vi "Write Core.vi"(8 "error in (no error)":errorcluster, 10 "Core":T1, 11 "ModuleAbstract in":refnum<class "ModuleAbstract.lvclass">) -> (0 "error out":errorcluster, 3 "ModuleAbstract out":refnum<class "ModuleAbstract.lvclass">)   [LabVIEW 2019, in "ModuleAbstract.lvlib" / "ModuleAbstract.lvclass"]
uses:
  ModuleAbstract.lvclass
  <vilib>/ActorFramework/Message Enqueuer/Message Enqueuer.lvclass
  ModuleAbstract.lvclass/ModuleAbstract.ctl
  Containers/ActorRefContainer/ActorRefContainer.lvclass/ActorRefContainer.ctl
  Containers/ActorRefContainer/ActorRefContainer.lvclass
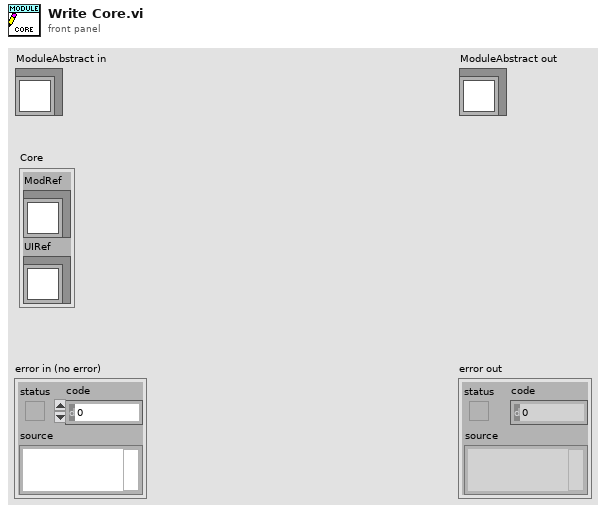
[diagram p1: front panel]
types:
  T1 = cluster{"ModRef":refnum<class "Message Enqueuer.lvclass">, "UIRef":refnum<class "Message Enqueuer.lvclass">}
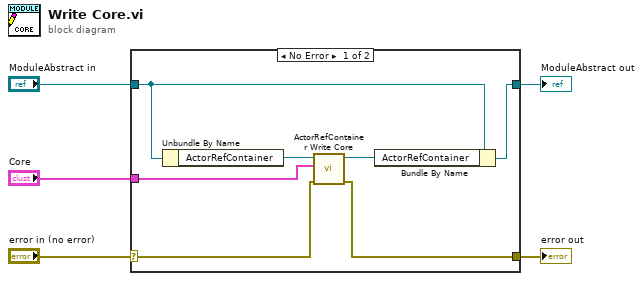
[diagram p0: block diagram]
diagram:
  n1 = case shown="No Error" "error in (no error)" {
    selector: "error in (no error)" -> [w8 w13]
    tunnel: [w7 w13] -> w4
    tunnel: [w12 w14] -> w2
    tunnel: "ModuleAbstract in" -> [w11 w14]
    tunnel: "Core" -> [w6 _]
    frame No Error {
      n2 = Unbundle By Name(w11) -> ("ActorRefContainer"=w10:refnum<class "ActorRefContainer.lvclass">)
      n3 = call "ActorRefContainer Write Core.vi"("error in (no error)"=w8, "Core"=w6, "ActorRefContainer in"=w10) -> ("error out"=w7:errorcluster, "ActorRefContainer out"=w9:refnum<class "ActorRefContainer.lvclass">)  [unwired: 7 in]
      n4 = Bundle By Name(cluster=w11, "ActorRefContainer"=w9) -> (w12:refnum<class "ModuleAbstract.lvclass">)
    }
    frame Error {
    }
  }
  "error out" <- w4
  "ModuleAbstract out" <- w2
